vi "Read_raw_inst_setup.vi"(0 "Setup file":string) -> (8 "Setup string":string, 10 "Ch & spans choices":T4(array[cluster]) {"D" format="%.2f"; "Ch No" min=0; "Sync Delay (ms)" min=-10.0 max=10.0 format="%.2f"}, 13 "PWA Data":T1, 14 "Number of Analogue instruments":i32=1, 16 "LDA data":enum16{"No LDA data", "Take LDA data"}(ring)=enum."Take LDA data", 17 "LDA set up":T3={"dimensions"=enum."2D", "Sampling Rate Hz"=0.1}, 19 "Synchronise Analogue channels with LDA":bool)   [LabVIEW 2017]
uses:
  Controls/Inst_type.ctl
  Controls/LDA_Setup.ctl
  Controls/PWA_Data.ctl
  Controls/Post_Process.ctl
  File/Setup_Filetype.ctl
  Controls/Trigger_Mode.ctl
  Controls/Tunnel_Coordinates.ctl
  Globals/Meas_global.vi
  Globals/LDA_meas_global_1.vi
  Globals/LDA_meas_global_2.vi
  Globals/Trav_pos_global.vi
panel:
  in  "Inst type":T2
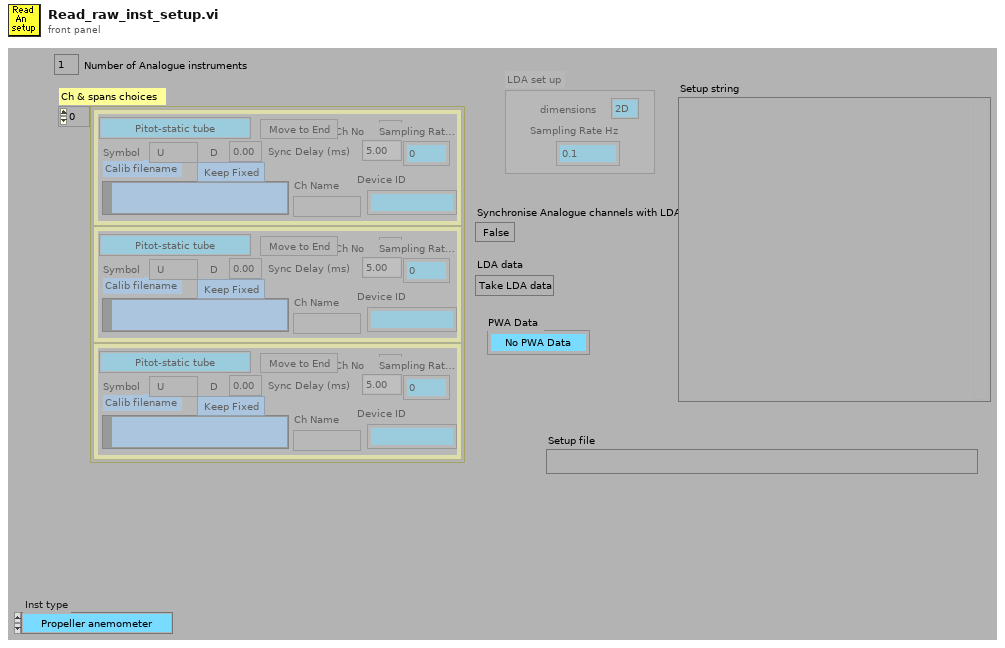
[diagram p1: front panel]
types:
  T1 = typedef "PWA_Data.ctl" = enum16{"No PWA Data", "One Ch PWA"}
  T2 = typedef "Inst_type.ctl" = enum16{"Propeller anemometer", "Raw voltage", "Pressure Transducer", "Pitot-static tube", "Preston tube", "Hot wire", "Cross wire 1", "Cross wire 2", "Generic Linear", "Generic Polynomial", "Generic BackPoly", "Fast FID", "Thermocouple", "Cold wire", "Pulsed Wire", "LDA Vel", "LDA Tran time", "LDA Arr time", "Microphone"}
  T3 = typedef "LDA_Setup.ctl" = cluster{"dimensions":enum16{"1D", "2D"}, "Sampling Rate Hz":dbl}
  T4 = cluster{"Ch No":i16, "Calib filename":path, "Inst type":T2, "Symbol":string, "Move channel":bool, "Use Latest":bool, "D":dbl, "Ch Name":string, "Sync Delay (ms)":dbl, "Device ID":string, "Sampling Rate Hz":dbl}[]
  T5 = typedef "Post_Process.ctl" = enum16{"Take New Data", "Post Process Raw Data File"}
  T6 = typedef "Setup_Filetype.ctl" = enum16{"Measurement Setups", "Calibration Setups", "General", "Results File Plotter Setups", "Speed Calib Tweaks"}
  T7 = typedef "Trigger_Mode.ctl" = enum16{"Free Running", "Start on Trigger", "Trigger Every Block", "Trigger Every Sample"}
  T8 = typedef "Tunnel_Coordinates.ctl" = enum16{"Work in Tunnel Coordinates", "Work in Model Coordinates"}
  T9 = cluster{"Ch No":i16, "Calib filename":path, "Inst type":T2, "Symbol":string, "Move channel":bool, "Use Latest":bool, "D":dbl, "Ch Name":string, "Sync Delay (ms)":dbl, "Device ID":string, "Sampling Rate Hz":dbl}
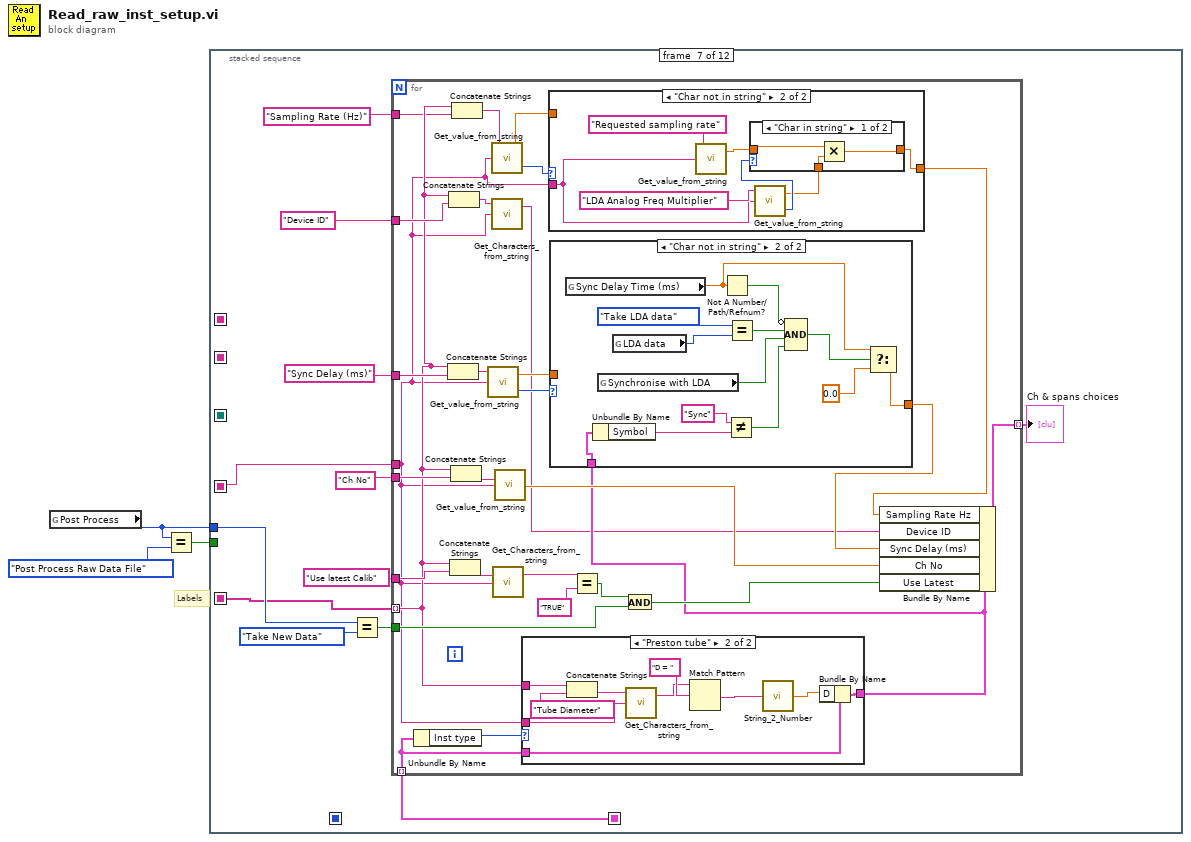
[diagram p0: block diagram]
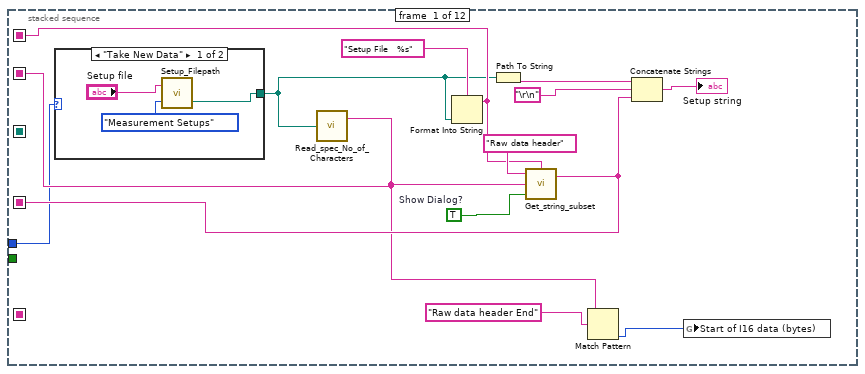
[diagram p2: hidden frame]
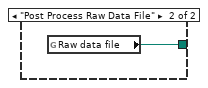
[diagram p3: hidden frame]
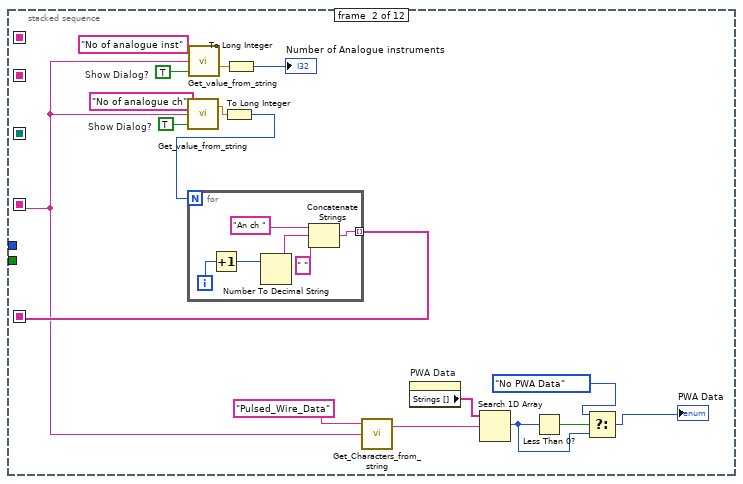
[diagram p4: hidden frame]
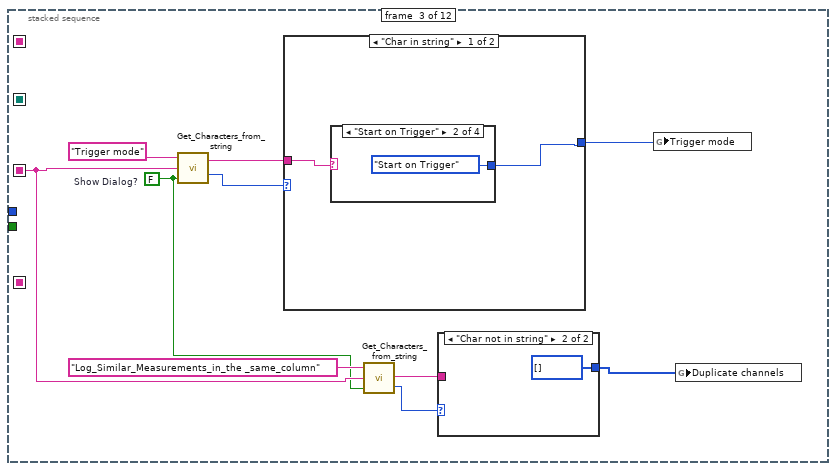
[diagram p5: hidden frame]
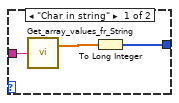
[diagram p6: hidden frame]
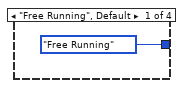
[diagram p7: hidden frame]
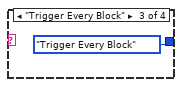
[diagram p8: hidden frame]
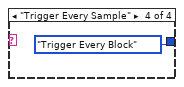
[diagram p9: hidden frame]
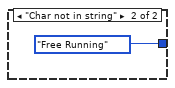
[diagram p10: hidden frame]
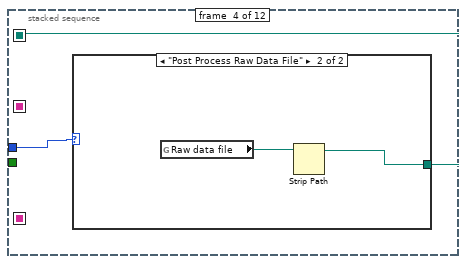
[diagram p11: hidden frame]
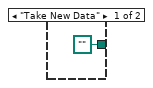
[diagram p12: hidden frame]
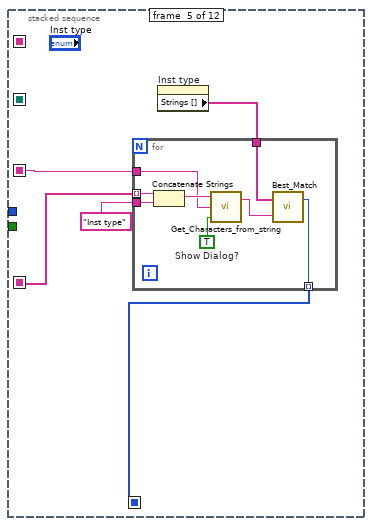
[diagram p13: hidden frame]
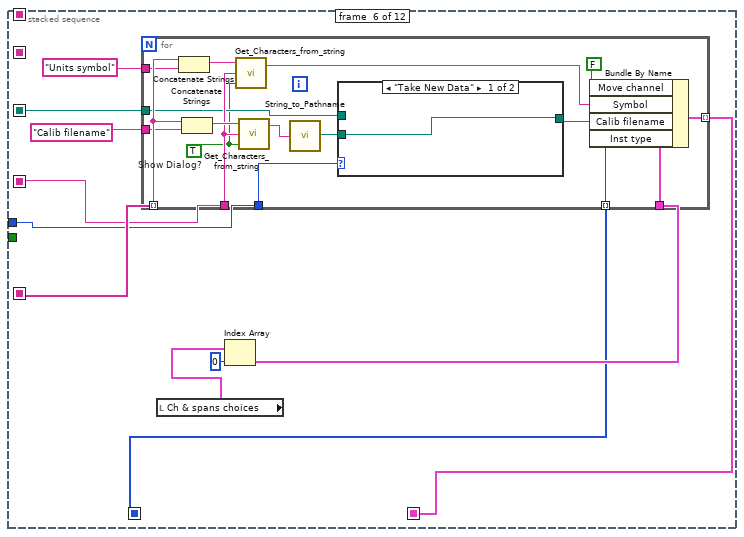
[diagram p14: hidden frame]
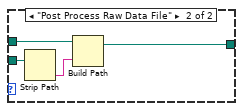
[diagram p15: hidden frame]
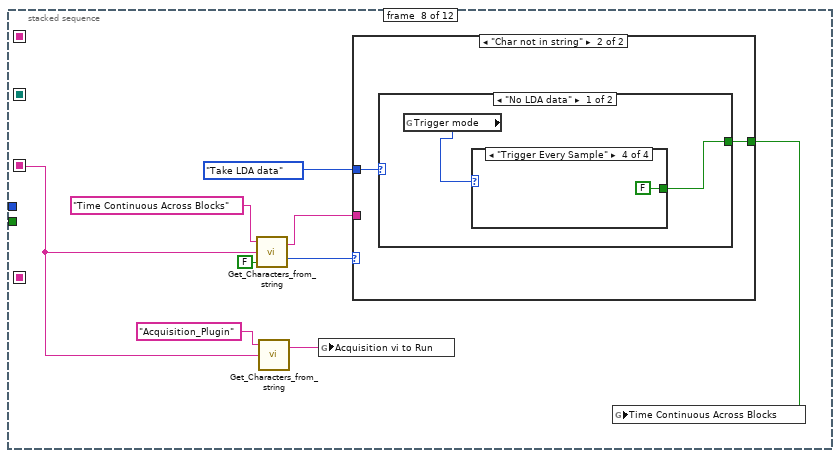
[diagram p20: hidden frame]
diagram:
  # "Labels"
  n1 = global read "Meas_global.vi" "Post Process"() -> (w1:T5)
  n2 = Equal?(x=w1, y=Post_Process."Post Process Raw Data File" ("Post Process")) -> (x = y?=w3:bool)
  n3 = stacked-sequence {
    seq-local: [w14 _ _ _ _ _ _ _ _ _ _ _] -> [_ w28 w48 _ w74 w84 w127 w200 w219 w222 w289 w314]
    seq-local: [_ w35 _ _ _ _ _ _ _ _ _ _] -> [_ _ _ _ w73 w93 w119 _ _ _ _ _]
    seq-local: [_ _ _ _ w70 _ _ _ _ _ _ _] -> [_ _ _ _ _ w87 _ _ _ _ _ _]
    seq-local: [_ _ _ _ _ w86 _ _ _ _ _ _] -> [_ _ _ _ _ _ w126 _ _ _ _ _]
    seq-local: [_ _ _ w66 _ _ _ _ _ _ _ _] -> [_ _ _ _ _ w85 _ _ _ _ _ _]
    seq-local: [w9 _ _ _ _ _ _ _ _ _ _ _] -> [_ _ _ _ _ _ _ _ _ _ _ w313]
    seq-local: [w6 _ _ _ _ _ _ _ _ _ _ _] -> [_ _ _ _ _ _ _ _ _ _ _ _]
    tunnel: w3 -> [_ _ _ _ _ _ _ _ _ _ _ w315]
    tunnel: w1 -> [w5 _ _ w65 _ w83 w120 _ _ _ _ _]
    frame #0 {
      w11 = TRUE  # Show Dialog?
      n4 = case shown="\"Take New Data\"" w5 {
        tunnel: [w17 w20] -> w4
        frame "Take New Data" {
          n5 = call "Setup_Filepath.vi"("Setup File Type"=Setup_Filetype."Measurement Setups", "Filename in"="Setup file") -> ("Filename Out"=w17:path)  [unwired: 1 out]
        }
        frame "Post Process Raw Data File" {
          n6 = global read "Meas_global.vi" "Raw data file"() -> (w20:path)
        }
      }
      n7 = call "Read_spec_No_of_Characters.vi"("Filename"=w4) -> ("character string"=w9:string)  [unwired: 1 out]
      n8 = Format Into String(format string="Setup File   %s", w4) -> (resulting string=w6:string)  [unwired: 2 in, 1 out]
      n9 = Path To String(path=w4) -> (string=w12:string)
      n10 = call "Get_string_subset.vi"("String Name"=w6, "Show Dialog?"=w11, "String to split"=w9, "File Label"="Raw data header") -> ("Output string"=w14:string)  [unwired: 1 out]
      n11 = Match Pattern(string=w9, regular expression="Raw data header End") -> (offset past match=w8:i32)  [unwired: 4 out]
      n12 = Concatenate Strings(w12, "\r\n", w14) -> (→"Setup string":string)
      n13 = global write "Meas_global.vi" "Start of I16 data (bytes)"(w8) -> ()
    }
    frame #1 {
      w29 = TRUE  # Show Dialog?
      w30 = TRUE  # Show Dialog?
      n14 = call "Get_value_from_string.vi"("Show Dialog?"=w30, "Input string"=w28, "Variable name"="No of analogue ch") -> ("Value"=w36:dbl)  [unwired: 1 out]
      n15 = call "Get_value_from_string.vi"("Show Dialog?"=w29, "Input string"=w28, "Variable name"="No of analogue inst") -> ("Value"=w33:dbl)  [unwired: 1 out]
      n16 = To Long Integer(number=w36) -> (32bit integer=w31:i32)
      n17 = for {
        N: w31 -> [_]
        tunnel: [w39] -> w35 mode=indexing
        i -> [w41]
        n18 = Increment(x=w41) -> (x+1=w40:i32)
        n19 = Number To Decimal String(number=w40) -> (decimal integer string=w43:string)  [unwired: 1 out]
        n20 = Concatenate Strings("An ch ", w43, " ") -> (w39:string)
      }
      n21 = To Long Integer(number=w33) -> (32bit integer=→"Number of Analogue instruments":i32)
      n22 = call "Get_Characters_from_string.vi"("Input string"=w28, "Variable name"="Pulsed_Wire_Data") -> ("Value"=w25:string)  [unwired: 1 in, 1 out]
      n23 = property on="PWA Data" class="Enum (strict)"() -> ("Strings []"=w26:string[])  [unwired: 2 in, 2 out]
      n24 = Search 1D Array(1D array=w26, element=w25) -> (index of element=w22:i32)  [unwired: 1 out]
      n25 = Less Than 0?(x=w22) -> (x < 0?=w24:bool)
      n26 = Select(t=PWA_Data."No PWA Data" ("PWA Data"), s=w24, f=w22) -> (s? t:f=→"PWA Data":i32)
    }
    frame #2 {
      w47 = FALSE  # Show Dialog?
      n27 = call "Get_Characters_from_string.vi"("Show Dialog?"=w47, "Input string"=w48, "Variable name"="Trigger mode") -> ("Status"=w52:enum16{"Char in string", "Char not in string"}, "Value"=w51:string)
      n28 = case shown="\"Char in string\"" w52 {
        tunnel: [w58 Trigger_Mode."Free Running" ("Trigger mode")] -> w50
        tunnel: w51 -> [w59 _]
        frame "Char in string" {
          n29 = case shown="\"Start on Trigger\"" w59 {
            tunnel: [Trigger_Mode."Free Running" ("Trigger mode") Trigger_Mode."Start on Trigger" ("Trigger mode") Trigger_Mode."Trigger Every Block" ("Trigger mode") Trigger_Mode."Trigger Every Block" ("Trigger mode")] -> w58
            frame "Free Running", Default {
            }
            frame "Start on Trigger" {
            }
            frame "Trigger Every Block" {
            }
            frame "Trigger Every Sample" {
            }
          }
        }
        frame "Char not in string" {
        }
      }
      n30 = call "Get_Characters_from_string.vi"("Show Dialog?"=w47, "Input string"=w48, "Variable name"="Log_Similar_Measurements_in_the _same_column") -> ("Status"=w44:enum16{"Char in string", "Char not in string"}, "Value"=w46:string)
      n31 = case shown="\"Char not in string\"" w44 {
        tunnel: w46 -> [w56 _]
        tunnel: [w54 i32[] []] -> w45
        frame "Char in string" {
          n32 = call "Get_array_values_fr_String.vi"("String Value"=w56) -> ("Numeric Array"=w55:dbl[])  [unwired: 1 out]
          n33 = To Long Integer(number=w55) -> (32bit integer=w54:i32[])
        }
        frame "Char not in string" {
        }
      }
      n34 = global write "Meas_global.vi" "Trigger mode"(w50) -> ()
      n35 = global write "Meas_global.vi" "Duplicate channels"(w45) -> ()
    }
    frame #3 {
      n36 = case shown="\"Post Process Raw Data File\"" w65 {
        tunnel: [path "" ("stripped path") w68] -> w66
        frame "Take New Data" {
        }
        frame "Post Process Raw Data File" {
          n37 = global read "Meas_global.vi" "Raw data file"() -> (w69:path)
          n38 = Strip Path(path=w69) -> (stripped path=w68:path)  [unwired: 1 out]
        }
      }
    }
    frame #4 {
      n39 = property on="Inst type" class="Enum (strict)"() -> ("Strings []"=w71:string[])  [unwired: 2 in, 2 out]
      n40 = for {
        tunnel: w74 -> [w81]
        tunnel: w71 -> [w77]
        tunnel: w73 -> [w80] mode=indexing
        tunnel: "Inst type" -> [w79]
        tunnel: [w75] -> w70 mode=indexing
        w78 = TRUE  # Show Dialog?
        n41 = Concatenate Strings(w80, w79) -> (w82:string)
        n42 = call "Get_Characters_from_string.vi"("Show Dialog?"=w78, "Input string"=w81, "Variable name"=w82) -> ("Value"=w76:string)  [unwired: 1 out]
        n43 = call "Best_Match.vi"("Input String"=w76, "String Options"=w77) -> ("index of element"=w75:i32)  [unwired: 1 out]
      }
    }
    frame #5 {
      n44 = local read "Ch & spans choices"() -> (w89:T4)
      n45 = Index Array(array=w89, index=0) -> (element=w88:T9)
      n46 = for {
        tunnel: w93 -> [w108] mode=indexing
        tunnel: "Calib filename" -> [w107]
        tunnel: "Units symbol" -> [w106]
        tunnel: w88 -> [w105]
        tunnel: w87 -> [w103] mode=indexing
        tunnel: [w102] -> w86 mode=indexing
        tunnel: w84 -> [w101]
        tunnel: w83 -> [w100]
        tunnel: w85 -> [w99]
        w96 = TRUE  # Show Dialog?
        n47 = Concatenate Strings(w108, w106) -> (w110:string)
        n48 = Concatenate Strings(w108, w107) -> (w109:string)
        n49 = call "Get_Characters_from_string.vi"("Show Dialog?"=w96, "Input string"=w101, "Variable name"=w110) -> ("Value"=w104:string)  [unwired: 1 out]
        n50 = call "Get_Characters_from_string.vi"("Show Dialog?"=w96, "Input string"=w101, "Variable name"=w109) -> ("Value"=w95:string)  [unwired: 1 out]
        n51 = call "String_to_Pathname.vi"("Input String"=w95) -> ("path"=w94:path)
        n52 = case shown="\"Take New Data\"" w100 {
          tunnel: w94 -> [w111 w115]
          tunnel: w99 -> [_ w112]
          tunnel: [w111 w113] -> w98
          frame "Take New Data" {
          }
          frame "Post Process Raw Data File" {
            n53 = Strip Path(path=w115) -> (name=w114:string)  [unwired: 1 out]
            n54 = Build Path(base path=w112, name or relative path=w114) -> (appended path=w113:path)
          }
        }
        n55 = Bundle By Name(cluster=w105, "Move channel"=FALSE, "Symbol"=w104, "Calib filename"=w98, "Inst type"=w103) -> (w102:T9)
      }
    }
    frame #6 {
      n56 = Equal?(x=w120, y=Post_Process."Take New Data" ("Post Process")) -> (x = y?=w118:bool)
      n57 = for {
        tunnel: "Sync Delay (ms)" -> [w156]
        tunnel: w126 -> [w143] mode=indexing
        tunnel: [w151] -> w125 mode=indexing
        tunnel: w127 -> [w128]
        tunnel: "Ch No" -> [w153]
        tunnel: "Use latest Calib" -> [w149]
        tunnel: w119 -> [w133] mode=indexing
        tunnel: w118 -> [w144]
        tunnel: "Device ID" -> [w135]
        tunnel: "Sampling Rate (Hz)" -> [w132]
        n58 = Unbundle By Name(w143) -> ("Inst type"=w145:T2)
        n59 = Concatenate Strings(w133, w156) -> (w155:string)
        n60 = Concatenate Strings(w133, w135) -> (w136:string)
        n61 = Concatenate Strings(w133, w149) -> (w150:string)
        n62 = Concatenate Strings(w133, w153) -> (w154:string)
        n63 = Concatenate Strings(w133, w132) -> (w134:string)
        n64 = call "Get_value_from_string.vi"("Input string"=w128, "Variable name"=w155) -> ("Status"=w141:enum16{"Char in string", "Char not in string"}, "Value"=w139:dbl)  [unwired: 1 in]
        n65 = call "Get_value_from_string.vi"("Input string"=w128, "Variable name"=w134) -> ("Status"=w131:enum16{"Char in string", "Char not in string"}, "Value"=w129:dbl)  [unwired: 1 in]
        n66 = call "Get_Characters_from_string.vi"("Input string"=w128, "Variable name"=w136) -> ("Value"=w137:string)  [unwired: 1 in, 1 out]
        n67 = call "Get_Characters_from_string.vi"("Input string"=w128, "Variable name"=w150) -> ("Value"=w148:string)  [unwired: 1 in, 1 out]
        n68 = call "Get_value_from_string.vi"("Input string"=w128, "Variable name"=w154) -> ("Value"=w152:dbl)  [unwired: 1 in, 1 out]
        n69 = case shown="\"Preston tube\"" w145 {
          tunnel: w133 -> [_ w193]
          tunnel: w128 -> [_ w188]
          tunnel: w143 -> [w183 w191]
          tunnel: [w183 w190] -> w138
          frame "Propeller anemometer", Default {
          }
          frame "Preston tube" {
            n70 = Concatenate Strings(w193, "Tube Diameter") -> (w189:string)
            n71 = call "Get_Characters_from_string.vi"("Input string"=w188, "Variable name"=w189) -> ("Value"=w186:string)  [unwired: 1 in, 1 out]
            n72 = Match Pattern(string=w186, regular expression="D = " ("String to match")) -> (after substring=w185:string)  [unwired: 4 out]
            n73 = call "String_2_Number.vi"("Value"=w185) -> ("Numeric"=w184:dbl)
            n74 = Bundle By Name(cluster=w191, "D"=w184) -> (w190:T9)
          }
        }
        n75 = case shown="\"Char not in string\"" w131 {
          tunnel: [w157 w160] -> w130
          tunnel: w129 -> [w157 _]
          tunnel: w128 -> [_ w162]
          frame "Char in string" {
          }
          frame "Char not in string" {
            n76 = call "Get_value_from_string.vi"("Input string"=w162, "Variable name"="Requested sampling rate") -> ("Value"=w159:dbl)  [unwired: 1 in, 1 out]
            n77 = call "Get_value_from_string.vi"("Input string"=w162, "Variable name"="LDA Analog Freq Multiplier") -> ("Status"=w161:enum16{"Char in string", "Char not in string"}, "Value"=w158:dbl)  [unwired: 1 in]
            n78 = case shown="\"Char in string\"" w161 {
              tunnel: [w165 w168] -> w160
              tunnel: w159 -> [w167 w168]
              tunnel: w158 -> [w166 _]
              frame "Char in string" {
                n79 = Multiply(x=w167, y=w166) -> (x*y=w165:dbl)
              }
              frame "Char not in string" {
              }
            }
          }
        }
        n80 = case shown="\"Char not in string\"" w141 {
          tunnel: [w169 w174] -> w140
          tunnel: w139 -> [w169 _]
          tunnel: w138 -> [_ w173]
          frame "Char in string" {
          }
          frame "Char not in string" {
            n81 = global read "LDA_meas_global_1.vi" "Sync Delay Time (ms)"() -> (w176:dbl)
            n82 = Unbundle By Name(w173) -> ("Symbol"=w172:string)
            n83 = global read "Meas_global.vi" "Synchronise with LDA"() -> (w180:bool)
            n84 = global read "Meas_global.vi" "LDA data"() -> (w181:enum16{"No LDA data", "Take LDA data"})
            n85 = Not A Number/Path/Refnum?(number/path/refnum=w176) -> (NaN/Path/Refnum?=w178:bool)
            n86 = Not Equal?(x="Sync", y=w172) -> (x != y?=w170:bool)
            n87 = Equal?(x=enum16{"No LDA data", "Take LDA data"}."Take LDA data", y=w181) -> (x = y?=w179:bool)
            n88 = Compound Arithmetic op=AND(invert w178, w179, w180, w170) -> (w177:bool)
            n89 = Select(t=w176, s=w177, f=0.0) -> (s? t:f=w174:dbl)
          }
        }
        n90 = Equal?(x=w148, y="TRUE") -> (x = y?=w146:bool)
        n91 = And(x=w146, y=w144) -> (x .and. y?=w142:bool)
        n92 = Bundle By Name(cluster=w138, "Sampling Rate Hz"=w130, "Device ID"=w137, "Sync Delay (ms)"=w140, "Ch No"=w152, "Use Latest"=w142) -> (w151:T9)
      }
      "Ch & spans choices" <- w125
    }
    frame #7 {
      n93 = call "Get_Characters_from_string.vi"("Show Dialog?"=FALSE, "Input string"=w200, "Variable name"="Time Continuous Across Blocks") -> ("Status"=w197:enum16{"Char in string", "Char not in string"}, "Value"=w195:string)
      n94 = call "Get_Characters_from_string.vi"("Input string"=w200, "Variable name"="Acquisition_Plugin") -> ("Value"=w201:string)  [unwired: 1 in, 1 out]
      n95 = global write "Meas_global.vi" "Acquisition vi to Run"(w201) -> ()
      n96 = case shown="\"Char not in string\"" w197 {
        tunnel: [w203 w207] -> w196
        tunnel: w195 -> [w205 _]
        tunnel: enum16{"No LDA data", "Take LDA data"}."Take LDA data" ("LDA data") -> [_ w206]
        frame "Char in string" {
          n97 = Equal?(x="TRUE", y=w205) -> (x = y?=w203:bool)
        }
        frame "Char not in string" {
          n98 = case shown="\"No LDA data\"" w206 {
            tunnel: [w208 FALSE ("Time Continuous Across Blocks")] -> w207
            frame "No LDA data" {
              n99 = global read "Meas_global.vi" "Trigger mode"() -> (w209:T7)
              n100 = case shown="\"Trigger Every Sample\"" w209 {
                tunnel: [TRUE TRUE FALSE FALSE] -> w208
                frame "Free Running" {
                }
                frame "Start on Trigger" {
                }
                frame "Trigger Every Block" {
                }
                frame "Trigger Every Sample" {
                }
              }
            }
            frame "Take LDA data" {
            }
          }
        }
      }
      n101 = global write "Meas_global.vi" "Time Continuous Across Blocks"(w196) -> ()
    }
    frame #8 {
      w216 = TRUE  # Show Dialog?
      n102 = property on="LDA data" class="Enum (strict)"() -> ("Strings []"=w215:string[])  [unwired: 2 in, 2 out]
      n103 = call "Get_Characters_from_string.vi"("Show Dialog?"=w216, "Input string"=w219, "Variable name"="LDA data" ("Label for characters")) -> ("Value"=w220:string)  [unwired: 1 out]
      n104 = Search 1D Array(1D array=w215, element=w220) -> (index of element=→"LDA data":i32)  [unwired: 1 out]
    }
    frame #9 {
      n105 = local read "LDA data"() -> (w221:enum16{"No LDA data", "Take LDA data"})
      n106 = case shown="\"Take LDA data\"" w221 {
        tunnel: w222 -> [_ w223]
        frame "No LDA data" {
        }
        frame "Take LDA data" {
          n107 = stacked-sequence {
            seq-local: [_ w229 _ _] -> [_ _ w259 _]
            seq-local: [_ _ w258 _] -> [_ _ _ w269]
            seq-local: [w225 _ _ _] -> [_ w231 _ _]
            tunnel: w223 -> [_ w228 _ w270]
            frame #0 {
              n108 = Build Array("LDA Dimensions", "LDA Req Sampling Rate Hz") -> (w225:string[])
            }
            frame #1 {
              n109 = local read "LDA set up"() -> (w230:T3)
              n110 = for {
                tunnel: w231 -> [w237] mode=indexing
                shift-right: [w234] -> w227
                shift-left: w230 -> [w235]
                tunnel: w228 -> [w232]
                n111 = call "Get_Characters_from_string.vi"("Input string"=w232, "Variable name"=w237) -> ("Status"=w236:enum16{"Char in string", "Char not in string"}, "Value"=w233:string)  [unwired: 1 in]
                n112 = case shown="\"Char in string\"" w236 {
                  tunnel: w237 -> [w241 _]
                  tunnel: w235 -> [w240 w257]
                  tunnel: [w239 w256] -> w234
                  tunnel: w233 -> [w238 _]
                  tunnel: w232 -> [_ w254]
                  frame "Char in string" {
                    n113 = case shown="\"LDA Dimensions\"" w241 {
                      tunnel: w240 -> [w245 w251 w252]
                      tunnel: [w244 w250 w252] -> w239
                      tunnel: w238 -> [w243 w249 _]
                      frame "LDA Dimensions" {
                        n114 = case shown="\"2D\", Default" w243 {
                          tunnel: [enum16{"1D", "2D"}."1D" ("Bundle Element") enum16{"1D", "2D"}."2D" ("Bundle Element")] -> w242
                          frame "1D" {
                          }
                          frame "2D", Default {
                          }
                        }
                        n115 = Bundle By Name(cluster=w245, "dimensions"=w242) -> (w244:T3)
                      }
                      frame "LDA Req Sampling Rate Hz" {
                        n116 = Fract/Exp String To Number(string=w249) -> (number=w248:dbl)  [unwired: 3 in, 1 out]
                        n117 = Bundle By Name(cluster=w251, "Sampling Rate Hz"=w248) -> (w250:T3)
                      }
                      frame "No Match", Default {
                      }
                    }
                  }
                  frame "Char not in string" {
                    n118 = call "Get_value_from_string.vi"("Input string"=w254, "Variable name"="Requested sampling rate") -> ("Value"=w253:dbl)  [unwired: 1 in, 1 out]
                    n119 = Bundle By Name(cluster=w257, "Sampling Rate Hz"=w253) -> (w256:T3)
                  }
                }
              }
              "LDA set up" <- w227
              n120 = Unbundle By Name(w227) -> ("dimensions"=w229:enum16{"1D", "2D"})
            }
            frame #2 {
              n121 = case shown="\"1D\"" w259 {
                tunnel: [1 2] -> w260
                frame "1D" {
                }
                frame "2D" {
                }
              }
              n122 = for {
                N: w260 -> [_]
                tunnel: [w262] -> w258 mode=indexing
                i -> [w264]
                n123 = Increment(x=w264) -> (x+1=w263:i32)
                n124 = Number To Decimal String(number=w263) -> (decimal integer string=w266:string)  [unwired: 1 out]
                n125 = Concatenate Strings("BSA ", w266, " ") -> (w262:string)
              }
            }
            frame #3 {
              n126 = for {
                tunnel: w270 -> [w272]
                tunnel: w269 -> [w273] mode=indexing
                i -> [w282]
                n127 = Concatenate Strings(w273, "Component") -> (w283:string)
                n128 = Concatenate Strings(w273, "Multiply Velocity by -1") -> (w277:string)
                n129 = Increment(x=w282) -> (x+1=w279:i32)
                n130 = call "Get_Characters_from_string.vi"("Input string"=w272, "Variable name"=w283) -> ("Value"=w280:string)  [unwired: 1 in, 1 out]
                n131 = call "Get_Characters_from_string.vi"("Show Dialog?"=FALSE, "Input string"=w272, "Variable name"=w277) -> ("Value"=w275:string)  [unwired: 1 out]
                n132 = Equal?(x=w275, y="TRUE") -> (x = y?=w271:bool)
                n133 = case shown="2" w279 {
                  tunnel: w280 -> [w285 w287]
                  tunnel: w271 -> [w284 w286]
                  frame 1, Default {
                    n134 = global write "LDA_meas_global_1.vi" "Vel Comp BSA1"(w285) -> ()
                    n135 = global write "LDA_meas_global_1.vi" "Multiply Velocity by -1"(w284) -> ()
                  }
                  frame 2 {
                    n136 = global write "LDA_meas_global_2.vi" "Vel Comp BSA2"(w287) -> ()
                    n137 = global write "LDA_meas_global_2.vi" "Multiply Velocity by -1"(w286) -> ()
                  }
                }
              }
            }
          }
        }
      }
    }
    frame #10 {
      n138 = Build Array("Synchronise with LDA") -> (w299:string[])
      n139 = Build Array("FALSE", "TRUE") -> (w296:string[])
      n140 = call "Get_value_from_string.vi"("Input string"=w289, "Variable name"="Sync Delay Time (ms)" ("Label for characters")) -> ("Status"=w291:enum16{"Char in string", "Char not in string"}, "Value"=w290:dbl)  [unwired: 1 in]
      n141 = case shown="\"Char not in string\"" w291 {
        tunnel: w290 -> [w301 _]
        tunnel: [w301 nan ("Value")] -> w288
        frame "Char in string" {
        }
        frame "Char not in string" {
        }
      }
      n142 = Build Array(FALSE, TRUE) -> (w293:bool[])
      n143 = for {
        tunnel: w289 -> [w310]
        tunnel: w299 -> [w306] mode=indexing
        tunnel: w296 -> [w305]
        tunnel: w293 -> [w304]
        i -> [w308]
        w303 = TRUE  # Show Dialog?
        n144 = call "Get_Characters_from_string.vi"("Show Dialog?"=w303, "Input string"=w310, "Variable name"=w306) -> ("Value"=w311:string)  [unwired: 1 out]
        n145 = Search 1D Array(1D array=w305, element=w311) -> (index of element=w309:i32)  [unwired: 1 out]
        n146 = Index Array(array=w304, index=w309) -> (element=w307:bool)
        n147 = case shown="1" w308 {
          tunnel: w307 -> [w312 _]
          frame 0, Default {
            "Synchronise Analogue channels with LDA" <- w312
          }
          frame 1 {
          }
        }
      }
      n148 = global write "LDA_meas_global_1.vi" "Sync Delay Time (ms)"(w288) -> ()
    }
    frame #11 {
      n149 = case shown="True" w315 {
        tunnel: w314 -> [_ w321]
        tunnel: w313 -> [_ w316]
        frame False {
        }
        frame True {
          w320 = FALSE  # Show Dialog?
          n150 = call "Get_Characters_from_string.vi"("Show Dialog?"=w320, "Input string"=w321, "Variable name"="Coordinate_System" ("Label for characters")) -> ("Status"=w319:enum16{"Char in string", "Char not in string"}, "Value"=w318:string)
          n151 = case shown="\"Char not in string\"" w319 {
            tunnel: w318 -> [w324 _]
            tunnel: [w323 w327] -> w317
            tunnel: w316 -> [_ w329]
            frame "Char in string" {
              n152 = case shown="\"Work in Model Coordinates\"" w324 {
                tunnel: [Tunnel_Coordinates."Work in Model Coordinates" ("Work in Tunnel Coordinates?") Tunnel_Coordinates."Work in Tunnel Coordinates" ("Work in Tunnel Coordinates?")] -> w323
                frame "Work in Model Coordinates" {
                }
                frame "Work in Tunnel Coordinates", Default {
                }
              }
            }
            frame "Char not in string" {
              n153 = Concatenate Strings("X Pos (Model)", "\t", "Y Pos (Model)") -> (w330:string)
              n154 = Match Pattern(string=w329, regular expression=w330) -> (offset past match=w328:i32)  [unwired: 4 out]
              n155 = case shown="-1" w328 {
                tunnel: [Tunnel_Coordinates."Work in Model Coordinates" ("Work in Tunnel Coordinates?") Tunnel_Coordinates."Work in Tunnel Coordinates" ("Work in Tunnel Coordinates?")] -> w327
                frame 0, Default {
                }
                frame -1 {
                }
              }
            }
          }
          n156 = global write "Trav_pos_global.vi" "Work in Tunnel Coordinates?"(w317) -> ()
        }
      }
    }
  }
